vi "Write Data Available.vi"(8 "error in (no error)":errorcluster, 10 "Data Available":refnum<notifier>, 11 "GUI In":refnum<class "GUI.lvclass">) -> (0 "error out":errorcluster, 3 "GUI Out":refnum<class "GUI.lvclass">)   [LabVIEW 2012, in "GUI.lvclass"]
uses:
  Reusable/GUI/GUI.lvclass
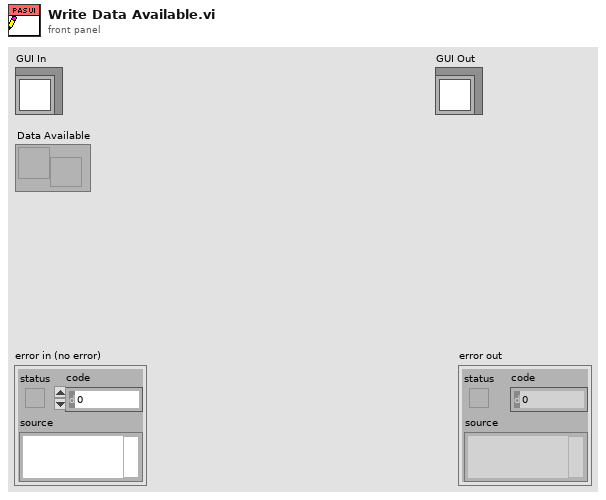
[diagram p1: front panel]
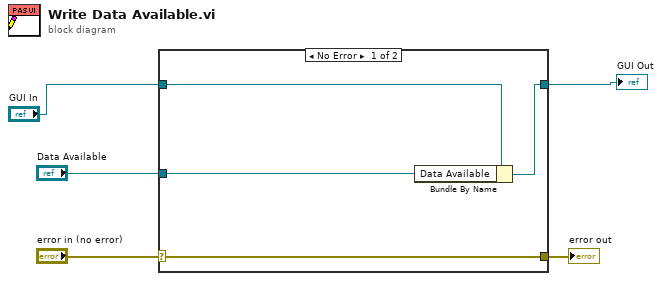
[diagram p0: block diagram]
diagram:
  n1 = case shown="No Error" "error in (no error)" {
    selector: "error in (no error)" -> [w9 w10]
    tunnel: [w9 w10] -> w4
    tunnel: [w7 w11] -> w1
    tunnel: "GUI In" -> [w8 w11]
    tunnel: "Data Available" -> [w6 _]
    frame No Error {
      n2 = Bundle By Name(cluster=w8, "Data Available"=w6) -> (w7:refnum<class "GUI.lvclass">)
    }
    frame Error {
    }
  }
  "error out" <- w4
  "GUI Out" <- w1
